vi "Edgertronic-get_saved_settings.vi"(3 "error in (no error)":errorcluster, 5 "URL":string="192.168.1.101") -> (0 "error out":errorcluster, 1 "Saved Settings:":T1={"Requested Genlock "="20140911165611", "Min Frame Clocks "="20140911165611", "Is Seq Clk Freq "="20140911165611", "Pretrigger Frames "="20140911165611", "Duration "="20140911165611", "Overclock "="20140911165611", "Requested Horizontal "="20140911165611", "Frames "="20140911165611", "Requested Pretrigger "="20140911165611", "Words per Frame "="20140911165611", "Buffer End "="20140911165611", "Clocks per Frame  "="20140911165611", "Requested Duration "="20140911165611", "Pretrigger "="20140911165611", "Post-trigger Frames "="20140911165611", "Vertical "="20140911165611", "Requested Vertical "="20140911165611", "Reqested Frame Rate "="20140911165611", "Frame Rate "="20140911165611", "Horizontal "="20140911165611", "Clocks per Exposure "="20140911165611", "Digital Gain "="20140911165611", "Exposure "="20140911165611", "Genlock "="20140911165611", "Analog Gain "="20140911165611", "Subsample "="20140911165611", "Requested Exposure "="20140911165611", "Iso "="20140911165611", "Requested Overclock "="20140911165611", "Requested Subsample "="20140911165611", "Requested Iso"="20140911165611", "Multishot"="20140911165611", "Requested Multishot"="20140911165611", "Monochrome"="20140911165611", "Requested mono"="20140911165611", "FPGA Temp"="20140911165611", "Is Temp"="20140911165611", "Posttrigger Duration"="20140911165611", "Pretrigger Duration"="20140911165611", "dacvrefadc"="20140911165611"})   [LabVIEW 2015]
doc: "This VI returns the values of the default settings."
uses:
  SettingsCtrl.ctl
panel:
  out "Connection Information:":string
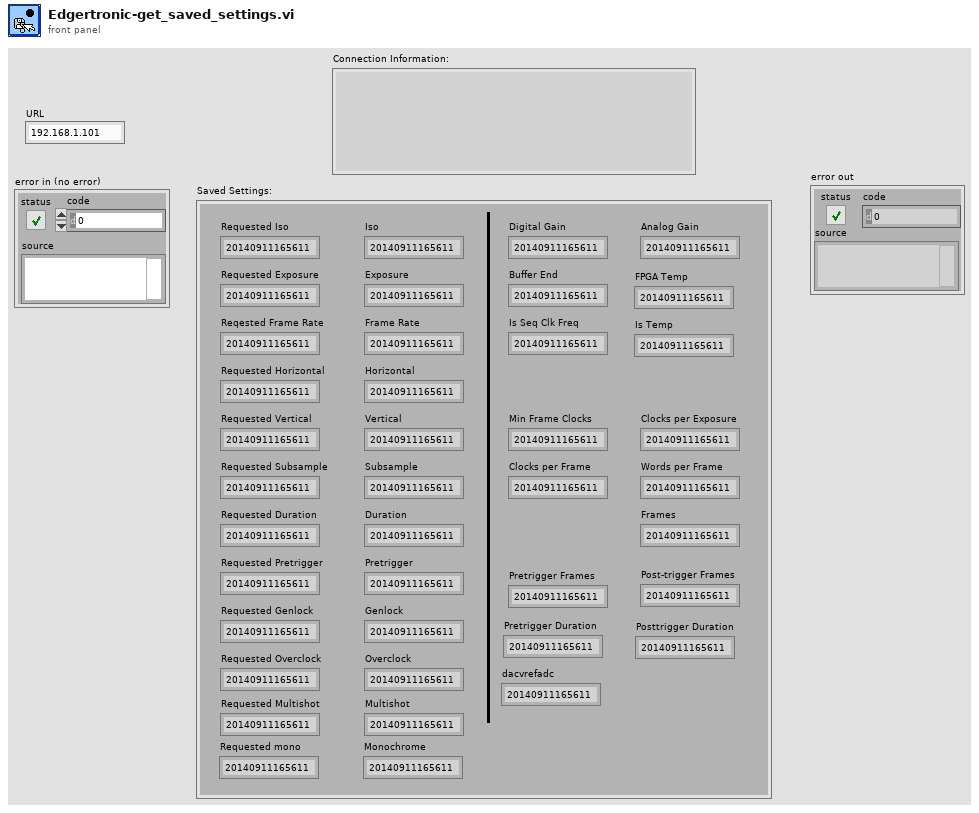
[diagram p1: front panel]
types:
  T1 = typedef "SettingsCtrl.ctl" = cluster{"Requested Genlock ":string, "Min Frame Clocks ":string, "Is Seq Clk Freq ":string, "Pretrigger Frames ":string, "Duration ":string, "Overclock ":string, "Requested Horizontal ":string, "Frames ":string, "Requested Pretrigger ":string, "Words per Frame ":string, "Buffer End ":string, "Clocks per Frame  ":string, "Requested Duration ":string, "Pretrigger ":string, "Post-trigger Frames ":string, "Vertical ":string, "Requested Vertical ":string, "Reqested Frame Rate ":string, "Frame Rate ":string, "Horizontal ":string, "Clocks per Exposure ":string, "Digital Gain ":string, "Exposure ":string, "Genlock ":string, "Analog Gain ":string, "Subsample ":string, "Requested Exposure ":string, "Iso ":string, "Requested Overclock ":string, "Requested Subsample ":string, "Requested Iso":string, "Multishot":string, "Requested Multishot":string, "Monochrome":string, "Requested mono":string, "FPGA Temp":string, "Is Temp":string, "Posttrigger Duration":string, "Pretrigger Duration":string, "dacvrefadc":string}
  T2 = cluster{"Requested Genlock ":string, "Min Frame Clocks ":string, "Is Seq Clk Freq ":string, "Pretrigger Frames ":string, "Duration ":string, "Overclock ":string, "Requested Horizontal ":string, "Frames ":string, "Requested Pretrigger ":string, "Words per Frame ":string, "Buffer End ":string, "Clocks per Frame  ":string, "Requested Duration ":string, "Pretrigger ":string, "Post-trigger Frames ":string, "Vertical ":string, "Requested Vertical ":string, "Reqested Frame Rate ":string, "Frame Rate ":string, "Horizontal ":string, "Clocks per Exposure ":string, "Digital Gain ":string, "Exposure ":string, "Genlock ":string, "Analog Gain ":string, "Subsample ":string, "Requested Exposure ":string, "Iso ":string, "Requested Overclock ":string, "Requested Subsample ":string, "Requested Iso":string, "Multishot":string, "Requested Multishot":string, "Monochrome":string, "Requested mono":string, "FPGA Temp":string, "Is Temp":string, "Posttrigger Duration":string, "Pretrigger Duration":string, "dacvrefadc":string}
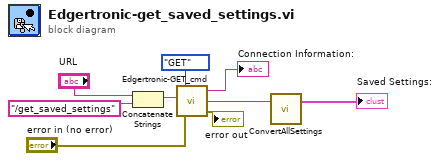
[diagram p0: block diagram]
diagram:
  n1 = Concatenate Strings("URL", "/get_saved_settings" ("GET Cmd")) -> (w4:string)
  n2 = call "Edgertronic-GET_cmd.vi"("error in (no error)"="error in (no error)", "URL"=w4, "Type"=enum16{"GET", "POST"}."GET") -> ("error out"=→"error out":errorcluster, "data"=w8:string, "Connection Info"=→"Connection Information:":string)  [unwired: 1 in]
  n3 = call "ConvertAllSettings.vi"("data"=w8) -> ("Saved Settings:"=→"Saved Settings:":T2)  [unwired: 2 in]
